vi "PixeLink MonitorAndSave.vi"(7 "Racine chemin de sauvegarde":path=path "Z:/Data Gas Experiments/Spring2019/sideview") -> ()   [LabVIEW 2014]
uses:
  <vilib>/addons/PixeLINK/Low Level Functions/ACQUISITION.llb/TDPU-Acquisition-StreamState.ctl
  <vilib>/addons/PixeLINK/Low Level Functions/CAMERA_FEATURES.llb/TDPU-CameraFeatures-FeatureIds.ctl
  <vilib>/addons/PixeLINK/Low Level Functions/CAMERA_FEATURES.llb/TDPU-CameraFeatures-FeatureFlags.ctl
  <vilib>/Platform/TimedLoop/XDataNode/timing_clust.ctl
  <vilib>/Platform/TimedLoop/XDataNode/nitl_modes.ctl
  <vilib>/Platform/TimedLoop/XDataNode/wakeup.ctl
  <vilib>/platform/TimedLoop/XDataNode/XDataNode.xnode
  <vilib>/Platform/TimedLoop/XDataNode/XDNodeRunTimeDep.lvlib
panel:
  in  "Colour/BW":bool
  in  "Dy":dbl format="%#_3g µm"
  in  "Dx":dbl format="%#_3g µm"
  in  "Calibration factor":dbl format="%#_g µm/px"
  out "Div":dbl
  out "Imager Serial #":u32[](array[numeric])
  in  "Chemins de sauvegarde":path[](array[path])
  in  "Bind Path to Camera":bool
  in  "Automatic\nfolder naming":bool=TRUE
  in  "Imager":u32(ring)=741003962 items=["High Res Side View"=95300230, "Focal Spot"=953000197, "Low Res Side View"=957000275]
  out "Error OUT 2":errorcluster
  out "Error OUT":errorcluster
  in  "Overwrite?":bool
  in  "Snap current Data":bool
  in  "Save Data":bool
  out "Warning":bool
  out "Message":string
  in  "Indice":u32
  in  "Nom du fichier":string="tir"
  in  "Mode de Sauvegarde":u16(ring)=1 items=["Manuel", "Automatique"]
  out "Captured Image":dbl[][](graph)
  out "Waiting for Trigger":bool
  in  "Continuous Grab":bool
  in  "Snap Next frame":bool
  out "Camera Handle":u32
  in  "Stop Grab\n(Insistez!)":bool
  in  "Trigger Type":enum16{"Free Running", "Software", "Hardware"}(ring)
  in  "Trigger Polarity":enum16{"Positive", "Negative"}(ring)
  in  "Refresh Trigger":bool
  in  "Exposure Time":dbl(slide) min=6.250873411772773e-05 max=10.0 scale=6.250873411772773e-05..10.0
  in  "stop":bool
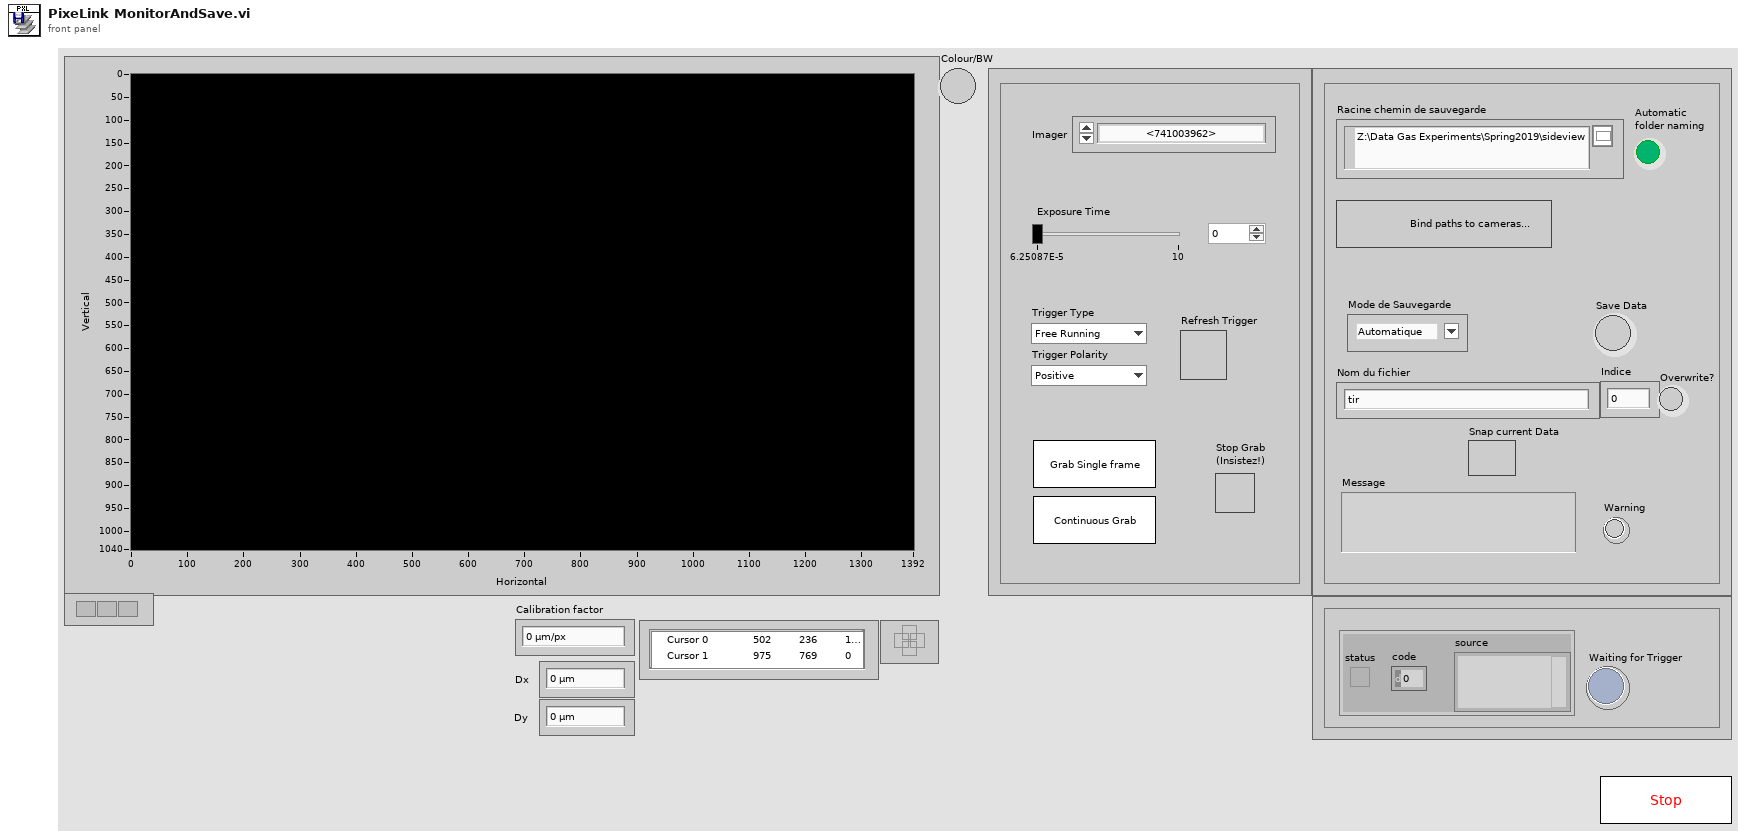
[diagram p1: front panel]
types:
  T1 = typedef "TDPU-Acquisition-StreamState.ctl" = u32
  T2 = typedef "TDPU-CameraFeatures-FeatureFlags.ctl" = u32
  T3 = typedef "TDPU-CameraFeatures-FeatureIds.ctl" = u32
  T4 = typedef "XDNodeRunTimeDep.lvlib/timing_clust.ctl" = cluster{"Expected End [f-1]":u64, "Actual End [f-1]":u64, "Finished Late? [f-1]":bool, "Expected End [i-1]":u64, "Actual End [i-1]":u64, "Finished Late? [i-1]":bool, "Expected Start [i]":u64, "Actual Start [i]":u64, "Expected Start [f]":u64, "Actual Start [f]":u64, "Source Name":string, "Structure Name":string, "Period":i64, "Deadline":i64, "Offset":i64, "Start":i64, "Priority":i32, "Timeout":i32, "Mode":T5, "Wakeup Reason":T6, "Error":errorcluster, "Source Type":string, "Secondary Source Type":string, "Global End Time":u64, "Global Start Time":u64, "Frame Duration":u64, "Iteration Duration":u64, "Assigned CPU":i32, "I/O Scan Engine Mode":u32}
  T5 = typedef "XDNodeRunTimeDep.lvlib/nitl_modes.ctl" = enum32{"No Change", "Process missed periods, maintain original phase", "Discard missed periods, maintain original phase", "Process missed periods, ignore original phase", "Discard missed periods, ignore original phase"}
  T6 = typedef "XDNodeRunTimeDep.lvlib/wakeup.ctl" = enum32{"Normal", "Aborted", "Asynchronous wakeup", "Timing source error", "Timed loop error", "Timeout"}
  T7 = typedef "LVStringsAndValuesArrayTypeDef_U32.ctl" = cluster{"String":string, "Value":u32}[]
  T8 = typedef "TDPU-Identification-Camera_Info.ctl" = cluster{"VendorName":string, "ModelName":string, "Description":string, "SerialNumber":string, "FirmwareVersion":string, "FPGAVersion":string, "CameraName":string}
  T9 = typedef "TDPU-Acquisition-Frame_Desc.ctl" = cluster{"uSize":u32, "fFrameTime":dbl, "uFrameNumber":u32, "Brightness":cluster{"fValue":dbl}, "AutoExposure":cluster{"fValue":dbl}, "Sharpness":cluster{"fValue":dbl}, "WhiteBalance":cluster{"fValue":dbl}, "Hue":cluster{"fValue":dbl}, "Saturation":cluster{"fValue":dbl}, "Gamma":cluster{"fValue":dbl}, "Shutter":cluster{"fValue":dbl}, "Gain":cluster{"fValue":dbl}, "Iris":cluster{"fValue":dbl}, "Focus":cluster{"fValue":dbl}, "Temperature":cluster{"fValue":dbl}, "Trigger":cluster{"fMode":dbl, "fType":dbl, "fPolarity":dbl, "fDelay":dbl, "fParameter":dbl}, "Zoom":cluster{"fValue":dbl}, "Pan":cluster{"fValue":dbl}, "Tilt":cluster{"fValue":dbl}, "OpticalFilter":cluster{"fValue":dbl}, "GPIO":cluster{"fMode":dbl[], "fPolarity":dbl[], "fParameter1":dbl[], "fParameter2":dbl[], "fParameter3":dbl[]}, "FrameRate":cluster{"fValue":dbl}, "ROI":cluster{"fLeft":dbl, "fTop":dbl, "fWidth":dbl, "fHeight":dbl}, "Flip":cluster{"fHorizontal":dbl, "fVertical":dbl}, "PixelAddressingValue":cluster{"fValue":dbl}, "PixelFormat":cluster{"fValue":dbl}, "ExtendedShutter":cluster{"fKneePoint":dbl[]}, "AutoROI":cluster{"fLeft":dbl, "fTop":dbl, "fWidth":dbl, "fHeight":dbl}, "WhiteShading":cluster{"fRedGain":dbl, "fGreenGain":dbl, "fBlueGain":dbl}, "Rotate":cluster{"fValue":dbl}, "PixelAddressingMode":cluster{"fValue":dbl}}
  T10 = typedef "LVPointDoubleTypeDef.ctl" = cluster{"Cursor X":dbl, "Cursor Y":dbl}
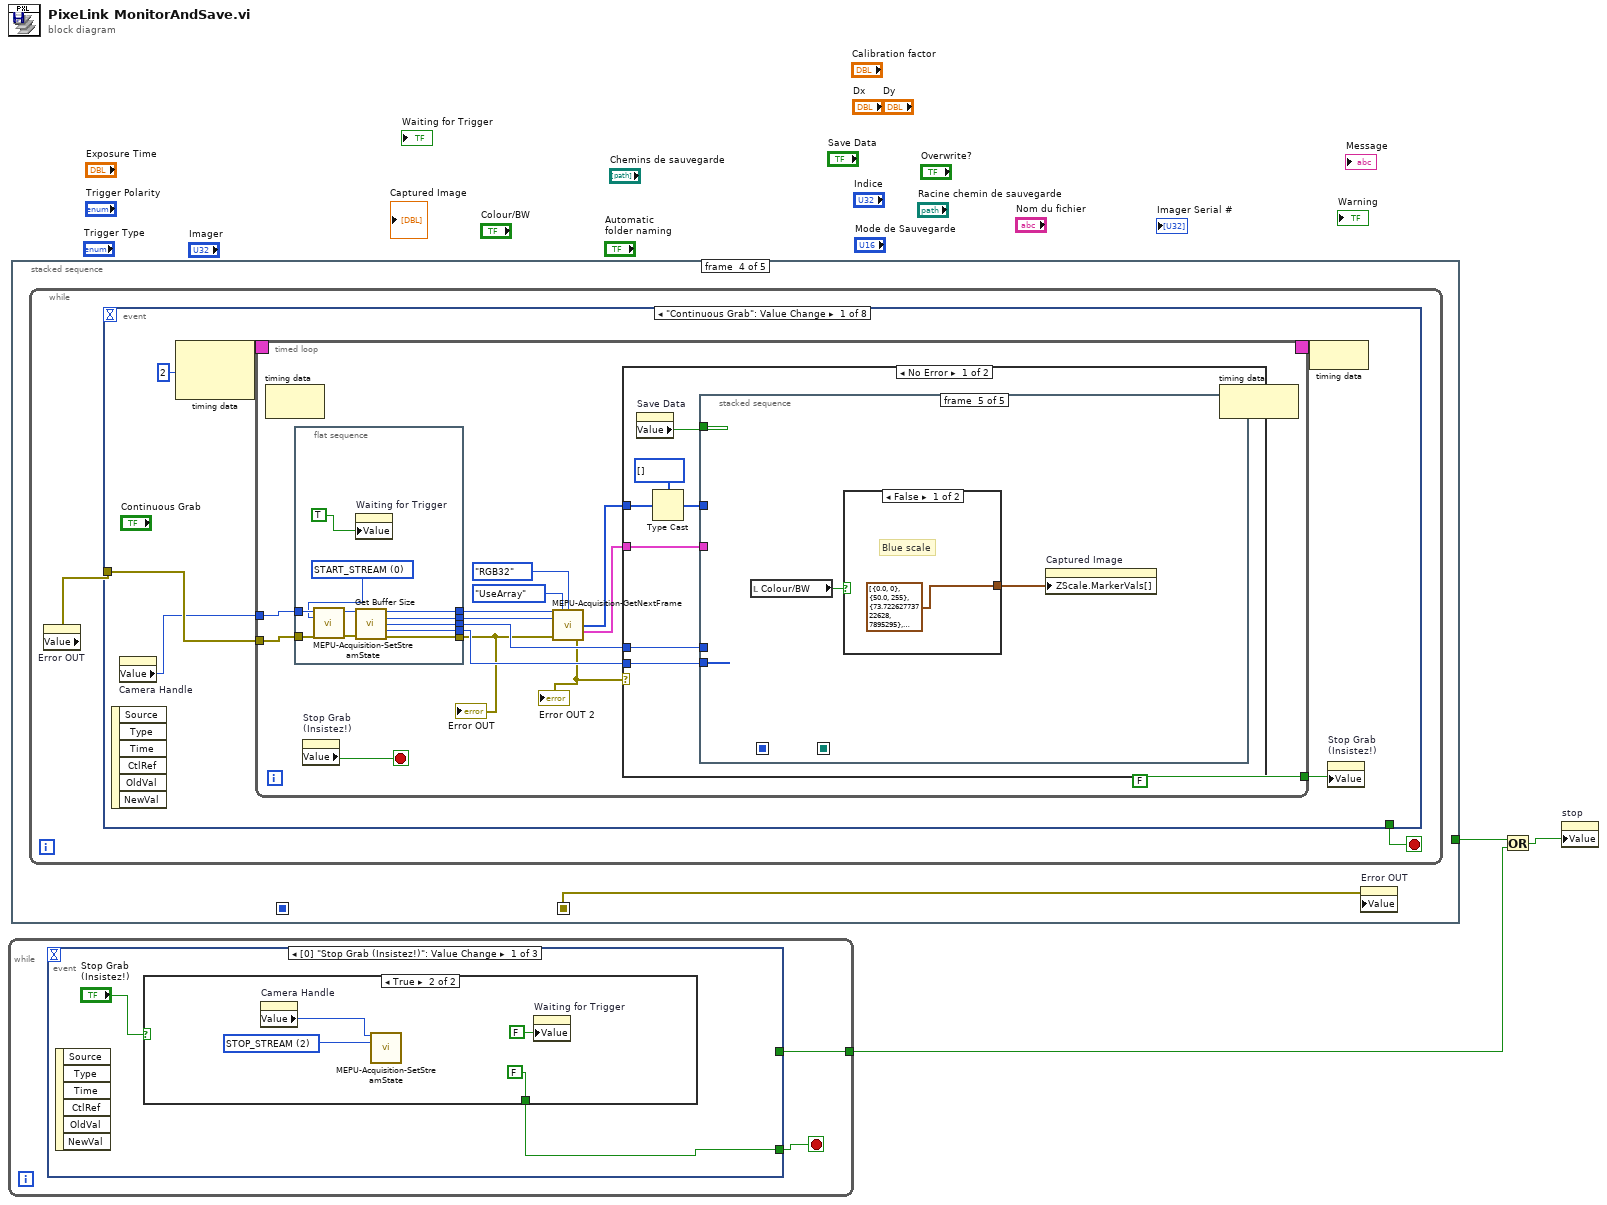
[diagram p0: block diagram]
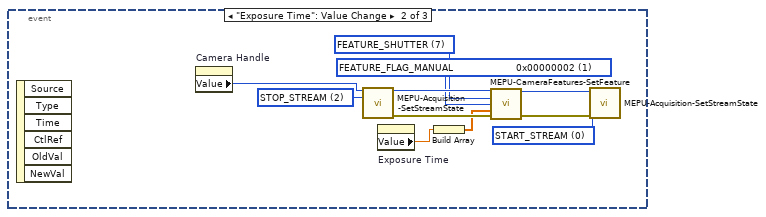
[diagram p3: hidden frame]
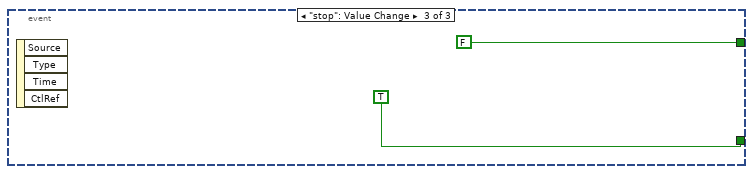
[diagram p4: hidden frame]
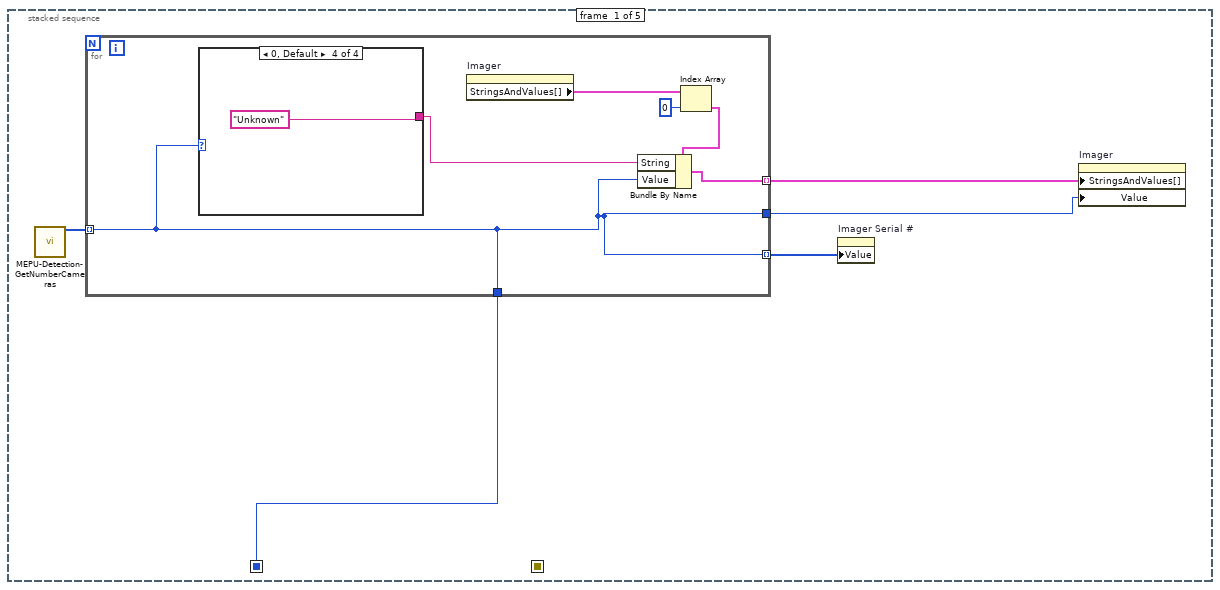
[diagram p5: hidden frame]
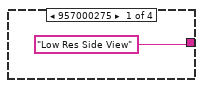
[diagram p6: hidden frame]
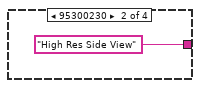
[diagram p7: hidden frame]
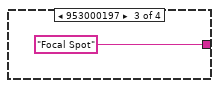
[diagram p8: hidden frame]
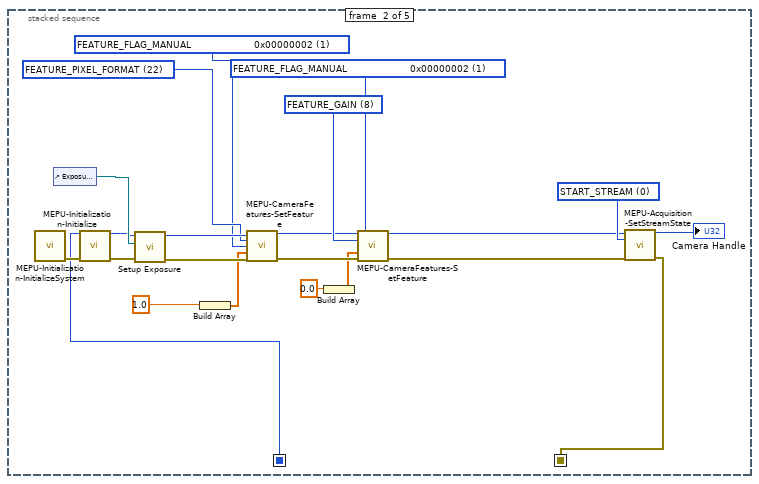
[diagram p9: hidden frame]
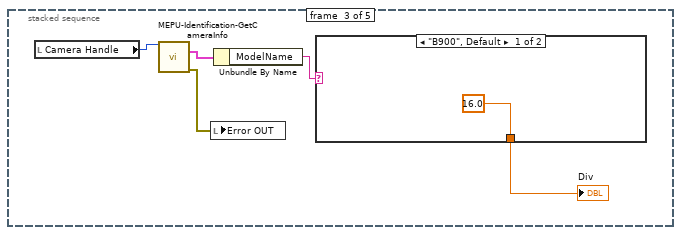
[diagram p10: hidden frame]
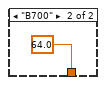
[diagram p11: hidden frame]
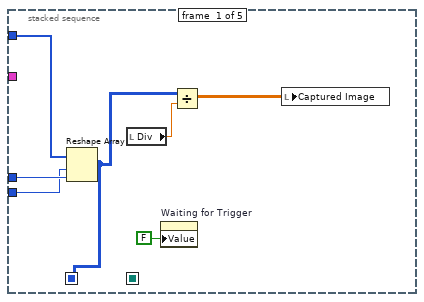
[diagram p12: hidden frame]
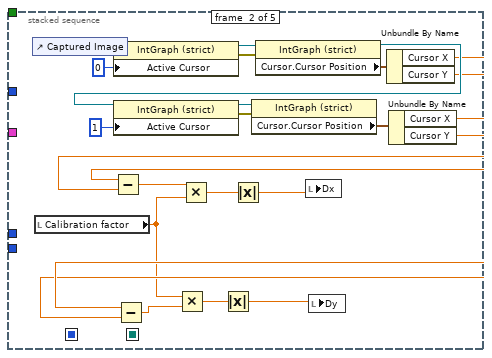
[diagram p13: hidden frame]
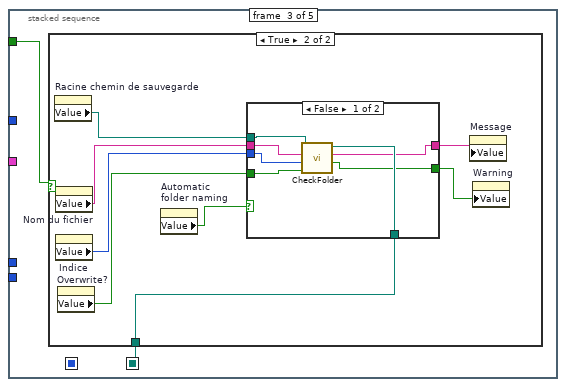
[diagram p14: hidden frame]
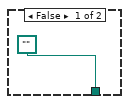
[diagram p15: hidden frame]
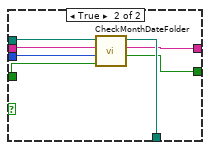
[diagram p16: hidden frame]
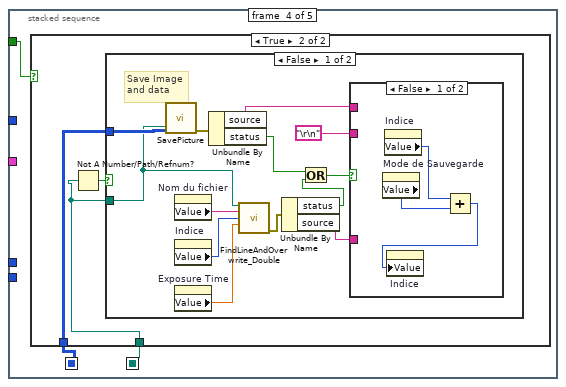
[diagram p17: hidden frame]
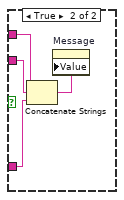
[diagram p19: hidden frame]
diagram:
  n1 = while {
    tunnel: [w4] -> w2
    stop <- w5 stop-if-true
    n2 = event shown="[0] \"Stop Grab (Insistez!)\": Value Change" {
      selector: _ -> [_ _ _]
      dyn-events: _ -> [_ _ _]
      timeout: _ -> [_ _ _]
      tunnel: [w6 _ TRUE] -> w5
      tunnel: [_ _ FALSE] -> w4
      event "Stop Grab\n(Insistez!)": Value Change {
        n3 = event-data() -> ()  [unwired: 1 in, 6 out]
        n4 = case shown="True" "Stop Grab\n(Insistez!)" {
          tunnel: [_ FALSE] -> w6
          frame False {
          }
          frame True {
            w11 = T1 2 items=["START_STREAM", "PAUSE_STREAM", "STOP_STREAM"] ("uStreamState IN")
            n5 = property on="Camera Handle" class="DigNum (strict)"() -> ("Value"=w9:u32)  [unwired: 2 in, 2 out]
            n6 = call <vilib>:"MEPU-Acquisition-SetStreamState.vi"("hCamera IN"=w9, "uStreamState IN"=w11) -> ()  [unwired: 12 in, 2 out]
            n7 = property on="Waiting for Trigger" class="Bool (strict)"("Value"=FALSE ("Waiting for Trigger")) -> ()  [unwired: 2 in, 2 out]
          }
        }
      }
      event "Exposure Time": Value Change {
        w22 = T1 0 items=["START_STREAM", "PAUSE_STREAM", "STOP_STREAM"] ("uStreamState IN")
        w21 = T1 2 items=["START_STREAM", "PAUSE_STREAM", "STOP_STREAM"] ("uStreamState IN")
        w14 = T2 1 items=["FEATURE_FLAG_PRESENCE                 0x00000001", "FEATURE_FLAG_MANUAL                     0x00000002", "FEATURE_FLAG_AUTO                         0x00000004", "FEATURE_FLAG_ONEPUSH                   0x00000008", "FEATURE_FLAG_OFF                            0x00000010", "FEATURE_FLAG_DESC_SUPPORTED    0x00000020", "FEATURE_FLAG_READ_ONLY               0x00000040"] ("uFlags IN")
        w13 = T3 7 items=["FEATURE_BRIGHTNESS", "FEATURE_EXPOSURE", "FEATURE_SHARPNESS", "FEATURE_WHITE_BAL", "FEATURE_HUE", "FEATURE_SATURATION", "FEATURE_GAMMA", "FEATURE_SHUTTER", "FEATURE_GAIN", "FEATURE_IRIS", "FEATURE_FOCUS", "FEATURE_TEMPERATURE", "FEATURE_TRIGGER", "FEATURE_ZOOM", "FEATURE_PAN", "FEATURE_TILT", "FEATURE_OPT_FILTER", "FEATURE_GPIO", "FEATURE_FRAME_RATE", "FEATURE_ROI", "FEATURE_FLIP", "FEATURE_PIXEL_ADDRESSING", "FEATURE_PIXEL_FORMAT", "FEATURE_EXTENDED_SHUTTER", "FEATURE_AUTO_ROI", "FEATURE_LOOKUP_TABLE", "FEATURE_MEMORY_CHANNEL", "FEATURE_WHITE_SHADING", "FEATURE_ROTATE", "FEATURE_IMAGER_CLK_DIVISOR", "FEATURE_TRIG_WITH_CNTRLD_LIGHT", "FEATURE_MAX_PIXEL_SIZE"] ("uFeatureId IN")
        n8 = event-data() -> ()  [unwired: 1 in, 6 out]
        n9 = property on="Camera Handle" class="DigNum (strict)"() -> ("Value"=w12:u32)  [unwired: 2 in, 2 out]
        n10 = call <vilib>:"MEPU-Acquisition-SetStreamState.vi"("hCamera IN"=w12, "uStreamState IN"=w21) -> ("hCamera OUT"=w17:u32, "Error OUT"=w20:errorcluster)  [unwired: 12 in]
        n11 = property on="Exposure Time" class="Slide (strict)"() -> ("Value"=w15:dbl)  [unwired: 2 in, 2 out]
        n12 = Build Array(w15) -> (w16:dbl[])
        n13 = call <vilib>:"MEPU-CameraFeatures-SetFeature.vi"("hCamera IN"=w17, "uFeatureId IN"=w13, "uFlags IN"=w14, "pParms IN"=w16, "Error IN"=w20) -> ("hCamera OUT"=w18:u32, "Error OUT"=w19:errorcluster)  [unwired: 9 out]
        n14 = call <vilib>:"MEPU-Acquisition-SetStreamState.vi"("hCamera IN"=w18, "uStreamState IN"=w22, "Error IN"=w19) -> ()  [unwired: 11 in, 2 out]
      }
      event "stop": Value Change {
        n15 = event-data() -> ()  [unwired: 1 in, 4 out]
      }
    }
  }
  n16 = stacked-sequence {
    seq-local: [_ w50 _ _ _] -> [_ _ _ w69 _]
    seq-local: [w28 _ _ _ _] -> [_ w40 _ _ _]
    tunnel: [_ _ _ _ TRUE] -> w3
    frame #0 {
      n17 = call <vilib>:"MEPU-Detection-GetNumberCameras.vi"() -> ("LV_SerialNumbers OUT"=w29:u32[])  [unwired: 13 in, 2 out]
      n18 = for {
        tunnel: w29 -> [w31] mode=indexing
        tunnel: [w35] -> w27 mode=indexing
        tunnel: [w31] -> w28
        tunnel: [w31] -> w26
        tunnel: [w31] -> w25 mode=indexing
        n19 = case shown="0, Default" w31 {
          tunnel: ["Low Res Side View" "High Res Side View" "Focal Spot" "Unknown"] -> w30
          frame 957000275 {
          }
          frame 95300230 {
          }
          frame 953000197 {
          }
          frame 0, Default {
          }
        }
        n20 = property on="Imager" class="Ring (strict)"() -> ("StringsAndValues[]"=w34:T7)  [unwired: 2 in, 2 out]
        n21 = Index Array(array=w34, index=0) -> (element=w32:cluster{"String":string, "Value":u32})
        n22 = Bundle By Name(cluster=w32, "String"=w30, "Value"=w31) -> (w35:cluster{"String":string, "Value":u32})
      }
      n23 = property on="Imager Serial #" class="Arr (strict)"("Value"=w25) -> ()  [unwired: 2 in, 2 out]
      n24 = property on="Imager" class="Ring (strict)"("StringsAndValues[]"=w27, "Value"=w26) -> ()  [unwired: 2 in, 2 out]
    }
    frame #1 {
      w45 = T2 1 items=["FEATURE_FLAG_PRESENCE                 0x00000001", "FEATURE_FLAG_MANUAL                     0x00000002", "FEATURE_FLAG_AUTO                         0x00000004", "FEATURE_FLAG_ONEPUSH                   0x00000008", "FEATURE_FLAG_OFF                            0x00000010", "FEATURE_FLAG_DESC_SUPPORTED    0x00000020", "FEATURE_FLAG_READ_ONLY               0x00000040"] ("uFlags IN")
      w44 = T3 8 items=["FEATURE_BRIGHTNESS", "FEATURE_EXPOSURE", "FEATURE_SHARPNESS", "FEATURE_WHITE_BAL", "FEATURE_HUE", "FEATURE_SATURATION", "FEATURE_GAMMA", "FEATURE_SHUTTER", "FEATURE_GAIN", "FEATURE_IRIS", "FEATURE_FOCUS", "FEATURE_TEMPERATURE", "FEATURE_TRIGGER", "FEATURE_ZOOM", "FEATURE_PAN", "FEATURE_TILT", "FEATURE_OPT_FILTER", "FEATURE_GPIO", "FEATURE_FRAME_RATE", "FEATURE_ROI", "FEATURE_FLIP", "FEATURE_PIXEL_ADDRESSING", "FEATURE_PIXEL_FORMAT", "FEATURE_EXTENDED_SHUTTER", "FEATURE_AUTO_ROI", "FEATURE_LOOKUP_TABLE", "FEATURE_MEMORY_CHANNEL", "FEATURE_WHITE_SHADING", "FEATURE_ROTATE", "FEATURE_IMAGER_CLK_DIVISOR", "FEATURE_TRIG_WITH_CNTRLD_LIGHT", "FEATURE_MAX_PIXEL_SIZE"] ("uFeatureId IN")
      w53 = T2 1 items=["FEATURE_FLAG_PRESENCE                 0x00000001", "FEATURE_FLAG_MANUAL                     0x00000002", "FEATURE_FLAG_AUTO                         0x00000004", "FEATURE_FLAG_ONEPUSH                   0x00000008", "FEATURE_FLAG_OFF                            0x00000010", "FEATURE_FLAG_DESC_SUPPORTED    0x00000020", "FEATURE_FLAG_READ_ONLY               0x00000040"] ("uFlags IN")
      w54 = T3 22 items=["FEATURE_BRIGHTNESS", "FEATURE_EXPOSURE", "FEATURE_SHARPNESS", "FEATURE_WHITE_BAL", "FEATURE_HUE", "FEATURE_SATURATION", "FEATURE_GAMMA", "FEATURE_SHUTTER", "FEATURE_GAIN", "FEATURE_IRIS", "FEATURE_FOCUS", "FEATURE_TEMPERATURE", "FEATURE_TRIGGER", "FEATURE_ZOOM", "FEATURE_PAN", "FEATURE_TILT", "FEATURE_OPT_FILTER", "FEATURE_GPIO", "FEATURE_FRAME_RATE", "FEATURE_ROI", "FEATURE_FLIP", "FEATURE_PIXEL_ADDRESSING", "FEATURE_PIXEL_FORMAT", "FEATURE_EXTENDED_SHUTTER", "FEATURE_AUTO_ROI", "FEATURE_LOOKUP_TABLE", "FEATURE_MEMORY_CHANNEL", "FEATURE_WHITE_SHADING", "FEATURE_ROTATE", "FEATURE_IMAGER_CLK_DIVISOR", "FEATURE_TRIG_WITH_CNTRLD_LIGHT", "FEATURE_MAX_PIXEL_SIZE"] ("uFeatureId IN")
      w60 = T1 0 items=["START_STREAM", "PAUSE_STREAM", "STOP_STREAM"] ("uStreamState IN")
      n25 = call <vilib>:"MEPU-Initialization-InitializeSystem.vi"() -> ("Error OUT"=w61:errorcluster)  [unwired: 15 in]
      n26 = control-ref of="Exposure Time"() -> (w59:refnum<vi>)
      n27 = call <vilib>:"MEPU-Initialization-Initialize.vi"("uSerialNumber IN"=w40, "Error IN"=w61) -> ("phCamera OUT"=w58:u32, "Error OUT"=w57:errorcluster)  [unwired: 11 in, 1 out]
      n28 = call "Setup Exposure.vi"("Error IN"=w57, "Shutter"=w59, "hCamera IN"=w58) -> ("Error OUT"=w56:errorcluster, "phCamera OUT"=w55:u32)  [unwired: 7 in]
      n29 = Build Array(1.0) -> (w51:dbl[])
      n30 = call <vilib>:"MEPU-CameraFeatures-SetFeature.vi"("hCamera IN"=w55, "uFeatureId IN"=w54, "uFlags IN"=w53, "pParms IN"=w51, "Error IN"=w56) -> ("hCamera OUT"=w43:u32, "Error OUT"=w48:errorcluster)  [unwired: 8 in, 1 out]
      n31 = Build Array(0.0) -> (w46:dbl[])
      n32 = call <vilib>:"MEPU-CameraFeatures-SetFeature.vi"("hCamera IN"=w43, "uFeatureId IN"=w44, "uFlags IN"=w45, "pParms IN"=w46, "Error IN"=w48) -> ("hCamera OUT"=w42:u32, "Error OUT"=w41:errorcluster)  [unwired: 8 in, 1 out]
      n33 = call <vilib>:"MEPU-Acquisition-SetStreamState.vi"("hCamera IN"=w42, "uStreamState IN"=w60, "Error IN"=w41) -> ("hCamera OUT"=→"Camera Handle":u32, "Error OUT"=w50:errorcluster)  [unwired: 11 in]
    }
    frame #2 {
      n34 = local read "Camera Handle"() -> (w66:u32)
      n35 = call <vilib>:"MEPU-Identification-GetCameraInfo.vi"("hCamera IN"=w66) -> ("pLVCameraInfo OUT"=w65:T8, "Error OUT"=w62:errorcluster)  [unwired: 12 in, 1 out]
      n36 = local write "Error OUT"(w62) -> ()
      n37 = Unbundle By Name(w65) -> ("ModelName"=w64:string)
      n38 = case shown="\"B900\", Default" w64 {
        tunnel: [16.0 64.0] -> w63
        frame "B900", Default {
        }
        frame "B700" {
        }
      }
      "Div" <- w63
    }
    frame #3 {
      n39 = while {
        stop <- w71 stop-if-true
        n40 = property on="Error OUT" class="Clust (strict)"() -> ("Value"=w70:errorcluster)  [unwired: 2 in, 2 out]
        n41 = event shown="[0] \"Continuous Grab\": Value Change" {
          selector: _ -> [_ _ _ _ _ _ _ _]
          dyn-events: _ -> [_ _ _ _ _ _ _ _]
          timeout: _ -> [_ _ _ _ _ _ _ _]
          tunnel: w70 -> [w77 _ _ _ w246 w264 _ _]
          tunnel: [_ _ _ TRUE _ _ _ _] -> w71
          event "Continuous Grab": Value Change {
            n42 = event-data() -> ()  [unwired: 1 in, 6 out]
            n43 = property on="Camera Handle" class="DigNum (strict)"() -> ("Value"=w72:u32)  [unwired: 2 in, 2 out]
            n44 = node-c288(i64 2 ("Period")) -> (w76:T4)  [unwired: 1 in]
            n45 = timed-loop {
              timing: w76 -> [_]
              timing-out: [_] -> w75
              tunnel: w72 -> [w91]
              tunnel: w77 -> [w85]
              tunnel: [FALSE] -> w73
              stop <- w82 stop-if-true
              n46 = node-c288() -> ()  [unwired: 1 in, 1 out]
              n47 = flat-sequence {
                tunnel: w91 -> [w183]
                tunnel: [w192] -> w90
                tunnel: [w191] -> w89
                tunnel: [w190] -> w80
                tunnel: w85 -> [w186]
                tunnel: [w189] -> w84
                tunnel: [w188] -> w83
                frame #0 {
                  w182 = T1 0 items=["START_STREAM", "PAUSE_STREAM", "STOP_STREAM"] ("uStreamState IN")
                  n48 = call <vilib>:"MEPU-Acquisition-SetStreamState.vi"("hCamera IN"=w183, "uStreamState IN"=w182, "Error IN"=w186) -> ("hCamera OUT"=w184:u32, "Error OUT"=w185:errorcluster)  [unwired: 11 in]
                  n49 = property on="Waiting for Trigger" class="Bool (strict)"("Value"=TRUE ("Waiting for Trigger")) -> ()  [unwired: 2 in, 2 out]
                  n50 = call "Get Buffer Size.vi"("phCamera IN"=w184, "Error IN"=w185) -> ("phCamera OUT"=w192:u32, "uBufferSize OUT"=w191:u32, "uWidth OUT"=w189:u32, "uHeight OUT"=w188:u32, "Error OUT"=w190:errorcluster)  [unwired: 8 in, 1 out]
                }
              }
              n51 = property on="Stop Grab\n(Insistez!)" class="Bool (strict)"() -> ("Value"=w82:bool)  [unwired: 2 in, 2 out]
              n52 = call <vilib>:"MEPU-Acquisition-GetNextFrame.vi"("hCamera IN"=w90, "Mode IN"=enum16{"UseArray", "UsePointer"}."UseArray", "OutputMode IN"=enum16{"Default", "RGB24", "RGB32"}."RGB32", "uBufferSize IN"=w89, "Error IN"=w80) -> ("Data OUT"=w86:u8[], "pDescriptor"=w78:T9, "Error OUT"=w79:errorcluster)  [unwired: 6 in, 2 out]
              "Error OUT 2" <- w79
              n53 = case shown="No Error" w79 {
                tunnel: w86 -> [w98 _]
                tunnel: w84 -> [w95 _]
                tunnel: w83 -> [w94 _]
                tunnel: w78 -> [w92 _]
                frame No Error {
                  n54 = property on="Save Data" class="Bool (strict)"() -> ("Value"=w93:bool)  [unwired: 2 in, 2 out]
                  n55 = Type Cast(type=u16[] [] ("Data OUT"), x=w98) -> (*(type *) &x=w96:u16[])
                  n56 = stacked-sequence {
                    seq-local: [_ _ w128 _ _] -> [_ _ _ w154 _]
                    seq-local: [w101 _ _ _ _] -> [_ _ _ w152 _]
                    tunnel: w96 -> [w105 _ _ _ _]
                    tunnel: w95 -> [w104 _ _ _ _]
                    tunnel: w94 -> [w103 _ _ _ _]
                    tunnel: w93 -> [_ _ w127 w153 _]
                    tunnel: w92 -> [_ _ _ _ _]
                    frame #0 {
                      n57 = Reshape Array(w105, w103, w104) -> (w101:u16[][])
                      n58 = local read "Div"() -> (w100:dbl)
                      n59 = property on="Waiting for Trigger" class="Bool (strict)"("Value"=FALSE ("Waiting for Trigger")) -> ()  [unwired: 2 in, 2 out]
                      n60 = Divide(x=w101, y=w100) -> (x/y=w99:dbl[][])
                      n61 = local write "Captured Image"(w99) -> ()
                    }
                    frame #1 {
                      n62 = control-ref of="Captured Image"() -> (w126:refnum<vi>)
                      n63 = local read "Calibration factor"() -> (w110:dbl)
                      n64 = property class="IntGraph (strict)"(reference=w126, "Active Cursor"=u32 0) -> (reference out=w124:refnum<vi>, error out=w123:errorcluster)  [unwired: 1 in]
                      n65 = property class="IntGraph (strict)"(reference=w124, error in=w123) -> (reference out=w122:refnum<vi>, "Cursor.Cursor Position"=w118:T10)  [unwired: 1 out]
                      n66 = property class="IntGraph (strict)"(reference=w122, "Active Cursor"=u32 1) -> (reference out=w120:refnum<vi>, error out=w119:errorcluster)  [unwired: 1 in]
                      n67 = property class="IntGraph (strict)"(reference=w120, error in=w119) -> ("Cursor.Cursor Position"=w117:T10)  [unwired: 2 out]
                      n68 = Unbundle By Name(w118) -> ("Cursor X"=w116:dbl, "Cursor Y"=w114:dbl)
                      n69 = Unbundle By Name(w117) -> ("Cursor X"=w115:dbl, "Cursor Y"=w113:dbl)
                      n70 = Subtract(x=w116, y=w115) -> (x-y=w111:dbl)
                      n71 = Subtract(x=w114, y=w113) -> (x-y=w112:dbl)
                      n72 = Multiply(x=w110, y=w112) -> (x*y=w108:dbl)
                      n73 = Multiply(x=w111, y=w110) -> (x*y=w109:dbl)
                      n74 = Absolute Value(x=w108) -> (abs(x)=w106:dbl)
                      n75 = Absolute Value(x=w109) -> (abs(x)=w107:dbl)
                      n76 = local write "Dx"(w107) -> ()
                      n77 = local write "Dy"(w106) -> ()
                    }
                    frame #2 {
                      n78 = case shown="True" w127 {
                        tunnel: [path "" ("File Path") w133] -> w128
                        frame False {
                        }
                        frame True {
                          n79 = property on="Racine chemin de sauvegarde" class="Path"() -> ("Value"=w134:path)  [unwired: 2 in, 2 out]
                          n80 = property on="Nom du fichier" class="Str"() -> ("Value"=w135:string)  [unwired: 2 in, 2 out]
                          n81 = property on="Indice" class="DigNum (strict)"() -> ("Value"=w136:u32)  [unwired: 2 in, 2 out]
                          n82 = property on="Overwrite?" class="Bool (strict)"() -> ("Value"=w137:bool)  [unwired: 2 in, 2 out]
                          n83 = property on="Automatic\nfolder naming" class="Bool (strict)"() -> ("Value"=w130:bool)  [unwired: 2 in, 2 out]
                          n84 = case shown="False" w130 {
                            tunnel: w137 -> [w142 w151]
                            tunnel: w136 -> [w143 w150]
                            tunnel: w135 -> [w144 w149]
                            tunnel: w134 -> [w141 w148]
                            tunnel: [w140 w147] -> w133
                            tunnel: [w139 w146] -> w132
                            tunnel: [w138 w145] -> w131
                            frame False {
                              n85 = call "CheckFolder.vi"("Overwrite?"=w142, "Index"=w143, "File Name"=w144, "Folder Path Control"=w141) -> ("Warning"=w138:bool, "Message"=w139:string, "File Path"=w140:path)  [unwired: 5 in]
                            }
                            frame True {
                              n86 = call "CheckMonthDateFolder.vi"("Overwrite?"=w151, "Index"=w150, "File Name"=w149, "Folder Path Control"=w148) -> ("Warning"=w145:bool, "Message"=w146:string, "File Path"=w147:path)  [unwired: 5 in]
                            }
                          }
                          n87 = property on="Message" class="Str"("Value"=w132) -> ()  [unwired: 2 in, 2 out]
                          n88 = property on="Warning" class="Bool (strict)"("Value"=w131) -> ()  [unwired: 2 in, 2 out]
                        }
                      }
                    }
                    frame #3 {
                      n89 = case shown="True" w153 {
                        tunnel: w154 -> [_ w156]
                        tunnel: w152 -> [_ w155]
                        frame False {
                        }
                        frame True {
                          n90 = Not A Number/Path/Refnum?(number/path/refnum=w156) -> (NaN/Path/Refnum?=w157:bool)
                          n91 = case shown="False" w157 {
                            tunnel: w156 -> [w161 _]
                            tunnel: w155 -> [w163 _]
                            frame False {
                              # "Save Image\nand data"
                              n92 = call "SavePicture.vi"("File Path"=w161, "Image Pixels (U16)"=w163) -> ("error out"=w169:errorcluster)  [unwired: 9 in]
                              n93 = property on="Nom du fichier" class="Str"() -> ("Value"=w160:string)  [unwired: 2 in, 2 out]
                              n94 = property on="Indice" class="DigNum (strict)"() -> ("Value"=w159:u32)  [unwired: 2 in, 2 out]
                              n95 = property on="Exposure Time" class="Slide (strict)"() -> ("Value"=w158:dbl)  [unwired: 2 in, 2 out]
                              n96 = Unbundle By Name(w169) -> ("source"=w166:string, "status"=w167:bool)
                              n97 = call "FindLineAndOverwrite_Double.vi"("Exposure path"=w161, "Name"=w160, "Index"=w159, "Exposure"=w158) -> ("error out"=w162:errorcluster)  [unwired: 11 in]
                              n98 = Unbundle By Name(w162) -> ("status"=w168:bool, "source"=w170:string)
                              n99 = Or(x=w167, y=w168) -> (x .or. y?=w165:bool)
                              n100 = case shown="False" w165 {
                                tunnel: w170 -> [_ w174]
                                tunnel: w166 -> [_ w177]
                                tunnel: "\r\n" -> [_ w175]
                                frame False {
                                n101 = property on="Mode de Sauvegarde" class="Ring (strict)"() -> ("Value"=w172:u16)  [unwired: 2 in, 2 out]
                                n102 = property on="Indice" class="DigNum (strict)"() -> ("Value"=w173:u32)  [unwired: 2 in, 2 out]
                                n103 = Add(x=w173, y=w172) -> (x+y=w171:u32)
                                n104 = property on="Indice" class="DigNum (strict)"("Value"=w171) -> ()  [unwired: 2 in, 2 out]
                                }
                                frame True {
                                n105 = Concatenate Strings(w177, w175, w174) -> (w176:string)
                                n106 = property on="Message" class="Str"("Value"=w176) -> ()  [unwired: 2 in, 2 out]
                                }
                              }
                            }
                            frame True {
                            }
                          }
                        }
                      }
                    }
                    frame #4 {
                      n107 = local read "Colour/BW"() -> (w179:bool)
                      n108 = case shown="False" w179 {
                        tunnel: [cluster{dbl, u32}[] [{0.0, 0}, {50.0, 255}, {73.72262773722628, 7895295}, {100.0, 16777215}] ("Z Scale.Marker Values[] 2") cluster{dbl, u32}[] [{0.0, 0}, {0.0, 0}, {0.0, 0}, {6.640316205533595, 786687}, {13.557312252964417, 1244928}, {27.391304347826086, 16776746}, {41.22529644268776, 16748842}, {54.940239043824675, 16646439}, {70.0, 16448250}, {70.0, 16448250}, {70.0, 16448250}, {70.0, 16448250}] ("Z Scale.Marker Values[]")] -> w178
                        frame False {
                          # "Blue scale"
                        }
                        frame True {
                          # "Colour scale"
                        }
                      }
                      n109 = property on="Captured Image" class="IntGraph (strict)"("ZScale.MarkerVals[]"=w178) -> ()  [unwired: 2 in, 2 out]
                    }
                  }
                }
                frame Error {
                }
              }
              n110 = node-c288() -> ()  [unwired: 1 in, 1 out]
              "Error OUT" <- w80
            }
            n111 = node-c288(w75) -> ()
            n112 = property on="Stop Grab\n(Insistez!)" class="Bool (strict)"("Value"=w73) -> ()  [unwired: 2 in, 2 out]
          }
          event "Imager": Value Change {
            n113 = event-data() -> ()  [unwired: 1 in, 6 out]
            n114 = flat-sequence {
              tunnel: [w205] -> w200
              tunnel: [w205] -> w199
              tunnel: w200 -> [w216]
              tunnel: w199 -> [w212]
              frame #0 {
                w202 = T1 2 items=["START_STREAM", "PAUSE_STREAM", "STOP_STREAM"] ("uStreamState IN")
                n115 = property on="Camera Handle" class="DigNum (strict)"() -> ("Value"=w201:u32)  [unwired: 2 in, 2 out]
                n116 = call <vilib>:"MEPU-Acquisition-SetStreamState.vi"("hCamera IN"=w201, "uStreamState IN"=w202) -> ("hCamera OUT"=w203:u32, "Error OUT"=w204:errorcluster)  [unwired: 12 in]
                n117 = call <vilib>:"MEPU-Initialization-Uninitialize.vi"("hCamera IN"=w203, "Error IN"=w204) -> ()  [unwired: 13 in, 1 out]
              }
              frame #1 {
                n118 = property on="Imager" class="Ring (strict)"() -> ("Strings []"=w210:string[], "RingText.Text"=w209:string, "StringsAndValues[]"=w208:T7)  [unwired: 2 in, 2 out]
                n119 = Search 1D Array(1D array=w210, element=w209) -> (index of element=w207:i32)  [unwired: 1 in]
                n120 = Index Array(array=w208, index=w207) -> (element=w206:cluster{"String":string, "Value":u32})
                n121 = Unbundle By Name(w206) -> ("Value"=w205:u32)
              }
              frame #2 {
                w233 = T1 0 items=["START_STREAM", "PAUSE_STREAM", "STOP_STREAM"] ("uStreamState IN")
                w230 = T3 8 items=["FEATURE_BRIGHTNESS", "FEATURE_EXPOSURE", "FEATURE_SHARPNESS", "FEATURE_WHITE_BAL", "FEATURE_HUE", "FEATURE_SATURATION", "FEATURE_GAMMA", "FEATURE_SHUTTER", "FEATURE_GAIN", "FEATURE_IRIS", "FEATURE_FOCUS", "FEATURE_TEMPERATURE", "FEATURE_TRIGGER", "FEATURE_ZOOM", "FEATURE_PAN", "FEATURE_TILT", "FEATURE_OPT_FILTER", "FEATURE_GPIO", "FEATURE_FRAME_RATE", "FEATURE_ROI", "FEATURE_FLIP", "FEATURE_PIXEL_ADDRESSING", "FEATURE_PIXEL_FORMAT", "FEATURE_EXTENDED_SHUTTER", "FEATURE_AUTO_ROI", "FEATURE_LOOKUP_TABLE", "FEATURE_MEMORY_CHANNEL", "FEATURE_WHITE_SHADING", "FEATURE_ROTATE", "FEATURE_IMAGER_CLK_DIVISOR", "FEATURE_TRIG_WITH_CNTRLD_LIGHT", "FEATURE_MAX_PIXEL_SIZE"] ("uFeatureId IN")
                w229 = T2 1 items=["FEATURE_FLAG_PRESENCE                 0x00000001", "FEATURE_FLAG_MANUAL                     0x00000002", "FEATURE_FLAG_AUTO                         0x00000004", "FEATURE_FLAG_ONEPUSH                   0x00000008", "FEATURE_FLAG_OFF                            0x00000010", "FEATURE_FLAG_DESC_SUPPORTED    0x00000020", "FEATURE_FLAG_READ_ONLY               0x00000040"] ("uFlags IN")
                w224 = T3 22 items=["FEATURE_BRIGHTNESS", "FEATURE_EXPOSURE", "FEATURE_SHARPNESS", "FEATURE_WHITE_BAL", "FEATURE_HUE", "FEATURE_SATURATION", "FEATURE_GAMMA", "FEATURE_SHUTTER", "FEATURE_GAIN", "FEATURE_IRIS", "FEATURE_FOCUS", "FEATURE_TEMPERATURE", "FEATURE_TRIGGER", "FEATURE_ZOOM", "FEATURE_PAN", "FEATURE_TILT", "FEATURE_OPT_FILTER", "FEATURE_GPIO", "FEATURE_FRAME_RATE", "FEATURE_ROI", "FEATURE_FLIP", "FEATURE_PIXEL_ADDRESSING", "FEATURE_PIXEL_FORMAT", "FEATURE_EXTENDED_SHUTTER", "FEATURE_AUTO_ROI", "FEATURE_LOOKUP_TABLE", "FEATURE_MEMORY_CHANNEL", "FEATURE_WHITE_SHADING", "FEATURE_ROTATE", "FEATURE_IMAGER_CLK_DIVISOR", "FEATURE_TRIG_WITH_CNTRLD_LIGHT", "FEATURE_MAX_PIXEL_SIZE"] ("uFeatureId IN")
                n122 = property on="Imager Serial #" class="Arr (strict)"() -> ("Value"=w213:u32[])  [unwired: 2 in, 2 out]
                n123 = property on="Chemins\n de sauvegarde" class="Arr (strict)"() -> ("Value"=w215:path[])  [unwired: 2 in, 2 out]
                n124 = Search 1D Array(1D array=w213, element=w212) -> (index of element=w211:i32)  [unwired: 1 in]
                n125 = Index Array(array=w215, index=w211) -> (element=w214:path)
                n126 = control-ref of="Exposure Time"() -> (w219:refnum<vi>)
                n127 = call <vilib>:"MEPU-Initialization-Initialize.vi"("uSerialNumber IN"=w216) -> ("phCamera OUT"=w218:u32, "Error OUT"=w217:errorcluster)  [unwired: 12 in, 1 out]
                n128 = Build Array(1.0) -> (w223:dbl[])
                n129 = call "Setup Exposure.vi"("Error IN"=w217, "Shutter"=w219, "hCamera IN"=w218) -> ("Error OUT"=w221:errorcluster, "phCamera OUT"=w220:u32)  [unwired: 7 in]
                n130 = property on="Racine chemin de sauvegarde" class="Path"("Value"=w214) -> ()  [unwired: 2 in, 2 out]
                n131 = call <vilib>:"MEPU-CameraFeatures-SetFeature.vi"("hCamera IN"=w220, "uFeatureId IN"=w224, "uFlags IN"=w229, "pParms IN"=w223, "Error IN"=w221) -> ("hCamera OUT"=w225:u32, "Error OUT"=w226:errorcluster)  [unwired: 8 in, 1 out]
                n132 = Build Array(0.0) -> (w228:dbl[])
                n133 = call <vilib>:"MEPU-CameraFeatures-SetFeature.vi"("hCamera IN"=w225, "uFeatureId IN"=w230, "uFlags IN"=w229, "pParms IN"=w228, "Error IN"=w226) -> ("hCamera OUT"=w231:u32, "Error OUT"=w232:errorcluster)  [unwired: 8 in, 1 out]
                n134 = call <vilib>:"MEPU-Acquisition-SetStreamState.vi"("hCamera IN"=w231, "uStreamState IN"=w233, "Error IN"=w232) -> ("hCamera OUT"=w234:u32)  [unwired: 11 in, 1 out]
                n135 = property on="Camera Handle" class="DigNum (strict)"("Value"=w234) -> ()  [unwired: 2 in, 2 out]
              }
            }
          }
          event "Trigger Polarity", "Trigger Type": Value Change {
            n136 = event-data() -> ()  [unwired: 1 in, 6 out]
            n137 = property on="Refresh Trigger" class="Bool"("Blinking"=TRUE) -> ()  [unwired: 2 in, 2 out]
          }
          event "stop": Value Change {
            n138 = event-data() -> ()  [unwired: 1 in, 6 out]
            n139 = property on="Refresh Trigger" class="Bool"("Blinking"=FALSE) -> ()  [unwired: 2 in, 2 out]
          }
          event "Refresh Trigger": Value Change {
            w240 = T1 2 items=["START_STREAM", "PAUSE_STREAM", "STOP_STREAM"] ("uStreamState IN")
            w241 = T1 0 items=["START_STREAM", "PAUSE_STREAM", "STOP_STREAM"] ("uStreamState IN")
            w255 = T2 1 items=["FEATURE_FLAG_PRESENCE                 0x00000001", "FEATURE_FLAG_MANUAL                     0x00000002", "FEATURE_FLAG_AUTO                         0x00000004", "FEATURE_FLAG_ONEPUSH                   0x00000008", "FEATURE_FLAG_OFF                            0x00000010", "FEATURE_FLAG_DESC_SUPPORTED    0x00000020", "FEATURE_FLAG_READ_ONLY               0x00000040"] ("uFlags IN")
            w256 = T3 12 items=["FEATURE_BRIGHTNESS", "FEATURE_EXPOSURE", "FEATURE_SHARPNESS", "FEATURE_WHITE_BAL", "FEATURE_HUE", "FEATURE_SATURATION", "FEATURE_GAMMA", "FEATURE_SHUTTER", "FEATURE_GAIN", "FEATURE_IRIS", "FEATURE_FOCUS", "FEATURE_TEMPERATURE", "FEATURE_TRIGGER", "FEATURE_ZOOM", "FEATURE_PAN", "FEATURE_TILT", "FEATURE_OPT_FILTER", "FEATURE_GPIO", "FEATURE_FRAME_RATE", "FEATURE_ROI", "FEATURE_FLIP", "FEATURE_PIXEL_ADDRESSING", "FEATURE_PIXEL_FORMAT", "FEATURE_EXTENDED_SHUTTER", "FEATURE_AUTO_ROI", "FEATURE_LOOKUP_TABLE", "FEATURE_MEMORY_CHANNEL", "FEATURE_WHITE_SHADING", "FEATURE_ROTATE", "FEATURE_IMAGER_CLK_DIVISOR", "FEATURE_TRIG_WITH_CNTRLD_LIGHT", "FEATURE_MAX_PIXEL_SIZE"] ("uFeatureId IN")
            n140 = event-data() -> ()  [unwired: 1 in, 6 out]
            n141 = property on="Camera Handle" class="DigNum (strict)"() -> ("Value"=w238:u32)  [unwired: 2 in, 2 out]
            n142 = property on="Refresh Trigger" class="Bool"("Blinking"=FALSE) -> ()  [unwired: 2 in, 2 out]
            n143 = property on="Trigger Polarity" class="Enum (strict)"() -> ("Value"=w251:enum16{"Positive", "Negative"})  [unwired: 2 in, 2 out]
            n144 = property on="Trigger Type" class="Enum (strict)"() -> ("Value"=w253:enum16{"Free Running", "Software", "Hardware"})  [unwired: 2 in, 2 out]
            n145 = To Double Precision Float(number=w251) -> (double precision float=w250:dbl)
            n146 = To Double Precision Float(number=w253) -> (double precision float=w252:dbl)
            n147 = Build Array(0.0 ("element"), w252, w250, 0.0 ("element"), 0.0 ("element")) -> (w247:dbl[])
            n148 = call <vilib>:"MEPU-Acquisition-SetStreamState.vi"("hCamera IN"=w238, "uStreamState IN"=w240, "Error IN"=w246) -> ("hCamera OUT"=w245:u32, "Error OUT"=w244:errorcluster)  [unwired: 11 in]
            n149 = call <vilib>:"MEPU-CameraFeatures-SetFeature.vi"("hCamera IN"=w245, "uFeatureId IN"=w256, "uFlags IN"=w255, "pParms IN"=w247, "Error IN"=w244) -> ("hCamera OUT"=w242:u32, "Error OUT"=w243:errorcluster)  [unwired: 9 out]
            n150 = call <vilib>:"MEPU-Acquisition-SetStreamState.vi"("hCamera IN"=w242, "uStreamState IN"=w241, "Error IN"=w243) -> ()  [unwired: 11 in, 2 out]
          }
          event "Snap Next frame": Value Change {
            w267 = T1 0 items=["START_STREAM", "PAUSE_STREAM", "STOP_STREAM"] ("uStreamState IN")
            n151 = event-data() -> ()  [unwired: 1 in, 6 out]
            n152 = flat-sequence {
              tunnel: w264 -> [w357]
              tunnel: [w357] -> w263
              frame #0 {
                n153 = property on="Waiting for Trigger" class="Bool (strict)"("Value"=TRUE ("Waiting for Trigger")) -> ()  [unwired: 2 in, 2 out]
              }
            }
            n154 = property on="Camera Handle" class="DigNum (strict)"() -> ("Value"=w257:u32)  [unwired: 2 in, 2 out]
            n155 = call <vilib>:"MEPU-Acquisition-SetStreamState.vi"("hCamera IN"=w257, "uStreamState IN"=w267, "Error IN"=w263) -> ("hCamera OUT"=w266:u32, "Error OUT"=w265:errorcluster)  [unwired: 11 in]
            n156 = call "Get Buffer Size.vi"("phCamera IN"=w266, "Error IN"=w265) -> ("phCamera OUT"=w271:u32, "uBufferSize OUT"=w269:u32, "uWidth OUT"=w260:u32, "uHeight OUT"=w259:u32, "Error OUT"=w270:errorcluster)  [unwired: 8 in, 1 out]
            n157 = call <vilib>:"MEPU-Acquisition-GetNextFrame.vi"("hCamera IN"=w271, "Mode IN"=enum16{"UseArray", "UsePointer"}."UseArray", "uBufferSize IN"=w269, "Error IN"=w270) -> ("Data OUT"=w262:u8[], "pDescriptor"=w258:T9, "Error OUT"=w261:errorcluster)  [unwired: 7 in, 2 out]
            n158 = property on="Error OUT 2" class="Clust (strict)"("Value"=w261) -> ()  [unwired: 2 in, 2 out]
            n159 = case shown="No Error" w261 {
              tunnel: w262 -> [w275 _]
              tunnel: w260 -> [w274 _]
              tunnel: w259 -> [w273 _]
              tunnel: w258 -> [w272 _]
              frame No Error {
                n160 = property on="Save Data" class="Bool (strict)"() -> ("Value"=w276:bool)  [unwired: 2 in, 2 out]
                n161 = Type Cast(type=u16[] [] ("Data OUT"), x=w275) -> (*(type *) &x=w277:u16[])
                n162 = stacked-sequence {
                  seq-local: [_ w287 _ _ _] -> [_ _ w308 _ _]
                  seq-local: [w280 _ _ _ _] -> [_ _ w306 _ _]
                  tunnel: w277 -> [w285 _ _ _ _]
                  tunnel: w276 -> [_ w286 w307 _ _]
                  tunnel: w274 -> [w283 _ _ _ _]
                  tunnel: w273 -> [w282 _ _ _ _]
                  tunnel: w272 -> [_ _ _ _ _]
                  frame #0 {
                    n163 = Reshape Array(w285, w282, w283) -> (w280:u16[][])
                    n164 = local read "Div"() -> (w281:dbl)
                    n165 = property on="Waiting for Trigger" class="Bool (strict)"("Value"=FALSE ("Waiting for Trigger")) -> ()  [unwired: 2 in, 2 out]
                    n166 = Divide(x=w280, y=w281) -> (x/y=w279:dbl[][])
                    n167 = property on="Captured Image" class="IntGraph (strict)"("Value"=w279) -> ()  [unwired: 2 in, 2 out]
                  }
                  frame #1 {
                    n168 = case shown="True" w286 {
                      tunnel: [path "" ("File Path") w291] -> w287
                      frame False {
                      }
                      frame True {
                        n169 = property on="Racine chemin de sauvegarde" class="Path"() -> ("Value"=w289:path)  [unwired: 2 in, 2 out]
                        n170 = property on="Automatic\nfolder naming" class="Bool (strict)"() -> ("Value"=w290:bool)  [unwired: 2 in, 2 out]
                        n171 = case shown="False" w290 {
                          tunnel: [w292 w299] -> w291
                          tunnel: w289 -> [w298 w300]
                          frame False {
                            n172 = property on="Nom du fichier" class="Str"() -> ("Value"=w295:string)  [unwired: 2 in, 2 out]
                            n173 = property on="Indice" class="DigNum (strict)"() -> ("Value"=w294:u32)  [unwired: 2 in, 2 out]
                            n174 = property on="Overwrite?" class="Bool (strict)"() -> ("Value"=w293:bool)  [unwired: 2 in, 2 out]
                            n175 = call "CheckFolder.vi"("Overwrite?"=w293, "Index"=w294, "File Name"=w295, "Folder Path Control"=w298) -> ("Warning"=w296:bool, "Message"=w297:string, "File Path"=w292:path)  [unwired: 5 in]
                            n176 = property on="Message" class="Str"("Value"=w297) -> ()  [unwired: 2 in, 2 out]
                            n177 = property on="Warning" class="Bool (strict)"("Value"=w296) -> ()  [unwired: 2 in, 2 out]
                          }
                          frame True {
                            n178 = property on="Nom du fichier" class="Str"() -> ("Value"=w303:string)  [unwired: 2 in, 2 out]
                            n179 = property on="Indice" class="DigNum (strict)"() -> ("Value"=w304:u32)  [unwired: 2 in, 2 out]
                            n180 = property on="Overwrite?" class="Bool (strict)"() -> ("Value"=w305:bool)  [unwired: 2 in, 2 out]
                            n181 = call "CheckMonthDateFolder.vi"("Overwrite?"=w305, "Index"=w304, "File Name"=w303, "Folder Path Control"=w300) -> ("Warning"=w301:bool, "Message"=w302:string, "File Path"=w299:path)  [unwired: 5 in]
                            n182 = property on="Warning" class="Bool (strict)"("Value"=w301) -> ()  [unwired: 2 in, 2 out]
                            n183 = property on="Message" class="Str"("Value"=w302) -> ()  [unwired: 2 in, 2 out]
                          }
                        }
                      }
                    }
                  }
                  frame #2 {
                    n184 = case shown="True" w307 {
                      tunnel: w308 -> [_ w310]
                      tunnel: w306 -> [_ w309]
                      frame False {
                      }
                      frame True {
                        n185 = Not A Number/Path/Refnum?(number/path/refnum=w310) -> (NaN/Path/Refnum?=w311:bool)
                        n186 = case shown="False" w311 {
                          tunnel: w310 -> [w315 _]
                          tunnel: w309 -> [w317 _]
                          frame False {
                            # "Save Image\nand data"
                            n187 = call "SavePicture.vi"("File Path"=w315, "Image Pixels (U16)"=w317) -> ("error out"=w323:errorcluster)  [unwired: 9 in]
                            n188 = property on="Nom du fichier" class="Str"() -> ("Value"=w314:string)  [unwired: 2 in, 2 out]
                            n189 = property on="Indice" class="DigNum (strict)"() -> ("Value"=w313:u32)  [unwired: 2 in, 2 out]
                            n190 = property on="Exposure Time" class="Slide (strict)"() -> ("Value"=w312:dbl)  [unwired: 2 in, 2 out]
                            n191 = Unbundle By Name(w323) -> ("source"=w320:string, "status"=w321:bool)
                            n192 = call "FindLineAndOverwrite_Double.vi"("Exposure path"=w315, "Name"=w314, "Index"=w313, "Exposure"=w312) -> ("error out"=w316:errorcluster)  [unwired: 11 in]
                            n193 = Unbundle By Name(w316) -> ("status"=w322:bool, "source"=w324:string)
                            n194 = Or(x=w321, y=w322) -> (x .or. y?=w319:bool)
                            n195 = case shown="False" w319 {
                              tunnel: w324 -> [_ w328]
                              tunnel: w320 -> [_ w331]
                              tunnel: "\r\n" -> [_ w329]
                              frame False {
                                n196 = property on="Mode de Sauvegarde" class="Ring (strict)"() -> ("Value"=w326:u16)  [unwired: 2 in, 2 out]
                                n197 = property on="Indice" class="DigNum (strict)"() -> ("Value"=w327:u32)  [unwired: 2 in, 2 out]
                                n198 = Add(x=w327, y=w326) -> (x+y=w325:u32)
                                n199 = property on="Indice" class="DigNum (strict)"("Value"=w325) -> ()  [unwired: 2 in, 2 out]
                              }
                              frame True {
                                n200 = Concatenate Strings(w331, w329, w328) -> (w330:string)
                                n201 = property on="Message" class="Str"("Value"=w330) -> ()  [unwired: 2 in, 2 out]
                              }
                            }
                          }
                          frame True {
                          }
                        }
                      }
                    }
                  }
                  frame #3 {
                    # "Check cursor positions"
                    n202 = control-ref of="Captured Image"() -> (w352:refnum<vi>)
                    n203 = local read "Calibration factor"() -> (w336:dbl)
                    n204 = property class="IntGraph (strict)"(reference=w352, "Active Cursor"=u32 0) -> (reference out=w350:refnum<vi>, error out=w349:errorcluster)  [unwired: 1 in]
                    n205 = property class="IntGraph (strict)"(reference=w350, error in=w349) -> (reference out=w348:refnum<vi>, "Cursor.Cursor Position"=w344:T10)  [unwired: 1 out]
                    n206 = property class="IntGraph (strict)"(reference=w348, "Active Cursor"=u32 1) -> (reference out=w346:refnum<vi>, error out=w345:errorcluster)  [unwired: 1 in]
                    n207 = property class="IntGraph (strict)"(reference=w346, error in=w345) -> ("Cursor.Cursor Position"=w343:T10)  [unwired: 2 out]
                    n208 = Unbundle By Name(w344) -> ("Cursor X"=w342:dbl, "Cursor Y"=w340:dbl)
                    n209 = Unbundle By Name(w343) -> ("Cursor X"=w341:dbl, "Cursor Y"=w339:dbl)
                    n210 = Subtract(x=w342, y=w341) -> (x-y=w337:dbl)
                    n211 = Subtract(x=w340, y=w339) -> (x-y=w338:dbl)
                    n212 = Multiply(x=w336, y=w338) -> (x*y=w334:dbl)
                    n213 = Multiply(x=w337, y=w336) -> (x*y=w335:dbl)
                    n214 = Absolute Value(x=w334) -> (abs(x)=w332:dbl)
                    n215 = Absolute Value(x=w335) -> (abs(x)=w333:dbl)
                    n216 = local write "Dx"(w333) -> ()
                    n217 = local write "Dy"(w332) -> ()
                  }
                  frame #4 {
                    n218 = local read "Colour/BW"() -> (w354:bool)
                    n219 = case shown="False" w354 {
                      tunnel: [cluster{dbl, u32}[] [{0.0, 0}, {50.0, 255}, {73.72262773722628, 7895295}, {100.0, 16777215}] ("Z Scale.Marker Values[] 2") cluster{dbl, u32}[] [{0.0, 0}, {0.0, 0}, {0.0, 0}, {6.640316205533595, 786687}, {13.557312252964417, 1244928}, {27.391304347826086, 16776746}, {41.22529644268776, 16748842}, {54.940239043824675, 16646439}, {70.0, 16448250}, {70.0, 16448250}, {70.0, 16448250}, {70.0, 16448250}] ("Z Scale.Marker Values[]")] -> w353
                      frame False {
                        # "Blue scale"
                      }
                      frame True {
                        # "Colour scale"
                      }
                    }
                    n220 = property on="Captured Image" class="IntGraph (strict)"("ZScale.MarkerVals[]"=w353) -> ()  [unwired: 2 in, 2 out]
                  }
                }
              }
              frame Error {
              }
            }
          }
          event "Bind Path to Camera": Value Change {
            n221 = event-data() -> ()  [unwired: 1 in, 6 out]
            n222 = property on="Imager" class="Ring (strict)"() -> ("StringsAndValues[]"=w364:T7)  [unwired: 2 in, 2 out]
            n223 = for {
              tunnel: w364 -> [w372] mode=indexing
              tunnel: [w367] -> w363 mode=indexing
              i -> [w368]
              n224 = Unbundle By Name(w372) -> ("String"=w371:string)
              n225 = Concatenate Strings("Choose path to save data\nfrom ", w371) -> (w369:string)
              n226 = Two Button Dialog(message=w369) -> (T button?=w367:bool)  [unwired: 2 in]
              n227 = case shown="True" w367 {
                tunnel: w368 -> [_ w374]
                frame False {
                }
                frame True {
                  n228 = call "File Dialog"() -> ("selected path"=w375:path, "error out"=w373:errorcluster)  [unwired: 12 in, 2 out]
                  n229 = case shown="No Error" w373 {
                    tunnel: w375 -> [w380 _]
                    tunnel: w374 -> [w377 _]
                    frame No Error {
                      n230 = property on="Chemins\n de sauvegarde" class="Arr (strict)"() -> ("Value"=w381:path[])  [unwired: 2 in, 2 out]
                      n231 = Array Size(array=w381) -> (size(s)=w379:i32)
                      n232 = Less Or Equal?(x=w379, y=w377) -> (x <= y?=w378:bool)
                      n233 = case shown="False" w378 {
                        tunnel: w381 -> [w385 w389]
                        tunnel: w380 -> [w383 w387]
                        tunnel: w377 -> [w384 w388]
                        tunnel: [w382 w386] -> w376
                        frame False {
                          n234 = Replace Array Subset(array=w385, new element=w383, index=w384) -> (w382:path[])
                        }
                        frame True {
                          n235 = Insert Into Array(array=w389, index=w388, new element=w387) -> (w386:path[])
                        }
                      }
                      n236 = property on="Chemins\n de sauvegarde" class="Arr (strict)"("Value"=w376) -> ()  [unwired: 2 in, 2 out]
                    }
                    frame Error {
                    }
                  }
                }
              }
            }
            n237 = property on="Imager" class="Ring (strict)"() -> ("Value"=w361:u32)  [unwired: 2 in, 2 out]
            n238 = property on="Imager Serial #" class="Arr (strict)"() -> ("Value"=w360:u32[])  [unwired: 2 in, 2 out]
            n239 = Search 1D Array(1D array=w360, element=w361) -> (index of element=w359:i32)  [unwired: 1 in]
            n240 = Index Array(array=w363, index=w359) -> (element=w362:bool)
            n241 = case shown="True" w362 {
              frame False {
              }
              frame True {
                # "If path to current cam data was changed, update on interface"
                n242 = property on="Chemins\n de sauvegarde" class="Arr (strict)"() -> ("Value"=w366:path[])  [unwired: 2 in, 2 out]
                n243 = Index Array(array=w366) -> (element=w365:path)  [unwired: 1 in]
                n244 = property on="Racine chemin de sauvegarde" class="Path"("Value"=w365) -> ()  [unwired: 2 in, 2 out]
              }
            }
          }
          event "Snap current Data": Value Change {
            n245 = event-data() -> ()  [unwired: 1 in, 6 out]
            n246 = stacked-sequence {
              seq-local: [w397 _] -> [_ w413]
              frame #0 {
                n247 = property on="Racine chemin de sauvegarde" class="Path"() -> ("Value"=w393:path)  [unwired: 2 in, 2 out]
                n248 = property on="Nom du fichier" class="Str"() -> ("Value"=w394:string)  [unwired: 2 in, 2 out]
                n249 = property on="Indice" class="DigNum (strict)"() -> ("Value"=w395:u32)  [unwired: 2 in, 2 out]
                n250 = property on="Overwrite?" class="Bool (strict)"() -> ("Value"=w396:bool)  [unwired: 2 in, 2 out]
                n251 = property on="Automatic\nfolder naming" class="Bool (strict)"() -> ("Value"=w390:bool)  [unwired: 2 in, 2 out]
                n252 = case shown="False" w390 {
                  tunnel: [w400 w411] -> w397
                  tunnel: w396 -> [w401 w410]
                  tunnel: w395 -> [w402 w409]
                  tunnel: w394 -> [w403 w408]
                  tunnel: w393 -> [w404 w407]
                  tunnel: [w399 w406] -> w392
                  tunnel: [w398 w405] -> w391
                  frame False {
                    n253 = call "CheckFolder.vi"("Overwrite?"=w401, "Index"=w402, "File Name"=w403, "Folder Path Control"=w404) -> ("Warning"=w398:bool, "Message"=w399:string, "File Path"=w400:path)  [unwired: 5 in]
                  }
                  frame True {
                    n254 = call "CheckMonthDateFolder.vi"("Overwrite?"=w410, "Index"=w409, "File Name"=w408, "Folder Path Control"=w407) -> ("Warning"=w405:bool, "Message"=w406:string, "File Path"=w411:path)  [unwired: 5 in]
                  }
                }
                n255 = property on="Warning" class="Bool (strict)"("Value"=w391) -> ()  [unwired: 2 in, 2 out]
                n256 = property on="Message" class="Str"("Value"=w392) -> ()  [unwired: 2 in, 2 out]
              }
              frame #1 {
                n257 = Not A Number/Path/Refnum?(number/path/refnum=w413) -> (NaN/Path/Refnum?=w412:bool)
                n258 = case shown="False" w412 {
                  tunnel: w413 -> [w418 _]
                  frame False {
                    # "Save Image\nand data"
                    n259 = property on="Captured Image" class="IntGraph (strict)"() -> ("Value"=w419:dbl[][])  [unwired: 2 in, 2 out]
                    n260 = call "SavePicture.vi"("File Path"=w418, "Image Pixels (U16)"=w419) -> ("error out"=w425:errorcluster)  [unwired: 9 in]
                    n261 = property on="Nom du fichier" class="Str"() -> ("Value"=w417:string)  [unwired: 2 in, 2 out]
                    n262 = property on="Indice" class="DigNum (strict)"() -> ("Value"=w416:u32)  [unwired: 2 in, 2 out]
                    n263 = property on="Exposure Time" class="Slide (strict)"() -> ("Value"=w415:dbl)  [unwired: 2 in, 2 out]
                    n264 = Unbundle By Name(w425) -> ("source"=w422:string, "status"=w423:bool)
                    n265 = call "FindLineAndOverwrite_Double.vi"("Exposure path"=w418, "Name"=w417, "Index"=w416, "Exposure"=w415) -> ("error out"=w414:errorcluster)  [unwired: 11 in]
                    n266 = Unbundle By Name(w414) -> ("status"=w424:bool, "source"=w426:string)
                    n267 = Or(x=w423, y=w424) -> (x .or. y?=w421:bool)
                    n268 = case shown="False" w421 {
                      tunnel: w426 -> [_ w430]
                      tunnel: w422 -> [_ w433]
                      tunnel: "\r\n" -> [_ w431]
                      frame False {
                        n269 = property on="Mode de Sauvegarde" class="Ring (strict)"() -> ("Value"=w428:u16)  [unwired: 2 in, 2 out]
                        n270 = property on="Indice" class="DigNum (strict)"() -> ("Value"=w429:u32)  [unwired: 2 in, 2 out]
                        n271 = Add(x=w429, y=w428) -> (x+y=w427:u32)
                        n272 = property on="Indice" class="DigNum (strict)"("Value"=w427) -> ()  [unwired: 2 in, 2 out]
                      }
                      frame True {
                        n273 = Concatenate Strings(w433, w431, w430) -> (w432:string)
                        n274 = property on="Message" class="Str"("Value"=w432) -> ()  [unwired: 2 in, 2 out]
                      }
                    }
                  }
                  frame True {
                  }
                }
              }
            }
          }
        }
      }
      n275 = property on="Error OUT" class="Clust (strict)"("Value"=w69) -> ()  [unwired: 2 in, 2 out]
    }
    frame #4 {
      w436 = T1 2 items=["START_STREAM", "PAUSE_STREAM", "STOP_STREAM"] ("uStreamState IN")
      # "Ignore errors here to ensure as\ncomplete a clean up as possible."
      n276 = property on="Camera Handle" class="DigNum (strict)"() -> ("Value"=w434:u32)  [unwired: 2 in, 2 out]
      n277 = call <vilib>:"MEPU-Acquisition-SetStreamState.vi"("hCamera IN"=w434, "uStreamState IN"=w436) -> ("hCamera OUT"=w438:u32)  [unwired: 12 in, 1 out]
      n278 = call <vilib>:"MEPU-Initialization-Uninitialize.vi"("hCamera IN"=w438) -> ("Error OUT"=w437:errorcluster)  [unwired: 14 in]
      n279 = stacked-sequence {
        tunnel: w437 -> [_]
        frame #0 {
          n280 = call <vilib>:"MEPU-Initialization-UninitializeSystem.vi"() -> ()  [unwired: 15 in, 1 out]
        }
      }
    }
  }
  n281 = Or(x=w3, y=w2) -> (x .or. y?=w1:bool)
  n282 = property on="stop" class="Bool (strict)"("Value"=w1) -> ()  [unwired: 2 in, 2 out]
